vi "Center-Aligned PWM Out - SCTL.vi"(2 "Low Pulse":u8, 3 "High Pulse":u8) -> (1 "Output":bool)   [LabVIEW 2016]
doc: "This VI will generate a PWM signal with the specified Duty Cycle and Period. Each period consists of an active state followed by an inactive state.\n\nThis VI is marked as re-entrant so that it it can be placed multiple times on the block diagram. Each time this VI is dropped on the block diagram, duplicate logic will be created in the FPGA.\n\nThis subVI was designed to work within a single cycle timed loop. If it is not used inside a single cycle timed loop, care should be taken to ensure that this VI is called at regular intervals. The period and duty cycle will be in terms of this interval period.\n\n<B>Inputs:</B>\n<B>Duty Cycle</B> - This is the active pulse width in terms of ticks if using in a single cycle timed loop or in terms of what ever interval it is called at. If the Duty cylce is equal to or greater than then the period the output will remain in it's active state. If the duty cycle is set to 0, the output will remain in it's inactive state. The duty cycle will only be reloaded at the end of each period.\n\n<B>Period</B> - This is the length of one complete Active/ Inactive pulse cycle. The period will only be reloaded at the end of each period. A period of 0 is equal to a period of 1.\n\n<B>Outputs:</B>\n<B>Output</B> - This is the output state of the PWM generator. A TRUE indicates the active state, a FALSE indicates the inactive state."
uses:
  <vilib>/rvi/Emulation/niFpgaSctlEmulationGetInTimedLoop.vi
  <vilib>/rvi/Emulation/niFpgaProcessEmulError.vi
panel:
  in  "Left Justified":bool=TRUE
  out "Curr. Duty Cycle":u8
  out "Curr. Period":u8
  out "Period Count":u8
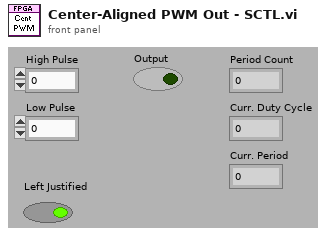
[diagram p1: front panel]
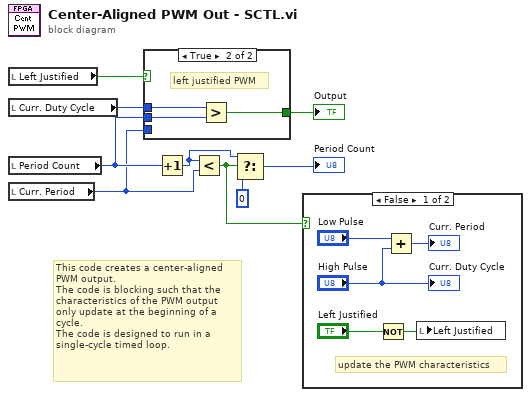
[diagram p0: block diagram]
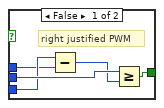
[diagram p2: hidden frame]
diagram:
  # "This code creates a center-aligned\nPWM output.  \nThe code is blocking such that the \ncharacteristics of the PWM output \nonly update at the beginning of a \ncycle.  \nThe code is designed to run in a \nsingle-cycle timed loop."
  n1 = local read "Left Justified"() -> (w1:bool)
  n2 = local read "Curr. Duty Cycle"() -> (w4:u8)
  n3 = local read "Period Count"() -> (w8:u8)
  n4 = local read "Curr. Period"() -> (w2:u8)
  n5 = case shown="True" w1 {
    tunnel: [w14 w17] -> w9
    tunnel: w8 -> [w13 w16]
    tunnel: w4 -> [w11 w15]
    tunnel: w2 -> [w12 _]
    frame False {
      # "right justified PWM"
      n6 = Subtract(x=w12, y=w11) -> (x-y=w10:u8)
      n7 = Greater Or Equal?(x=w13, y=w10) -> (x >= y?=w14:bool)
    }
    frame True {
      # "left justified PWM"
      n8 = Greater?(x=w15, y=w16) -> (0:w17:bool)
    }
  }
  "Output" <- w9
  n9 = Increment(x=w8) -> (x+1=w7:u8)
  n10 = Less?(x=w7, y=w2) -> (x < y?=w3:bool)
  n11 = Select(t=w7, s=w3, f=u8 0 ("t")) -> (s? t:f=→"Period Count":u8)
  n12 = case shown="False" w3 {
    frame False {
      # "update the PWM characteristics"
      n13 = Not(x="Left Justified") -> (.not. x?=w18:bool)
      n14 = Add(x="Low Pulse", y="High Pulse") -> (x+y=→"Curr. Period":u8)
      n15 = local write "Left Justified"(w18) -> ()
      "Curr. Duty Cycle" <- "High Pulse"
    }
    frame True {
    }
  }
